vi "Map to Table.vi"(0 "Data":T1, 5 "error in":errorcluster) -> (14 "Value":string[][](array[string]), 19 "error out":errorcluster)   [LabVIEW 2024]
uses:
  Type Def/Data.ctl
panel:
  # "Connector Pane"
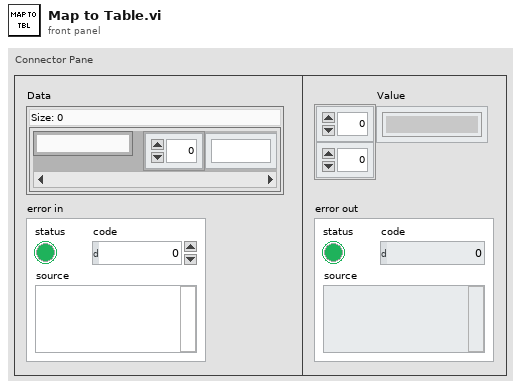
[diagram p1: front panel]
types:
  T1 = typedef "Data.ctl" = map{string, dbl[]}
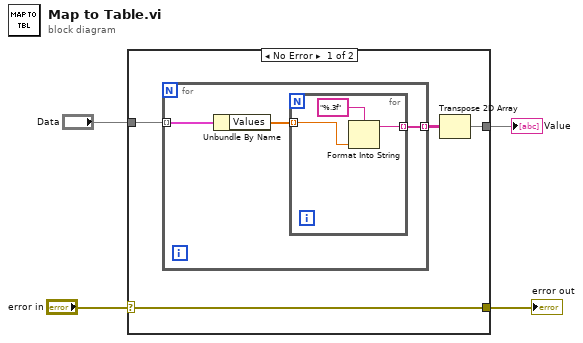
[diagram p0: block diagram]
diagram:
  n1 = case shown="No Error" "error in" {
    selector: "error in" -> [w6 w15]
    tunnel: [w6 w15] -> w3
    tunnel: "Data" -> [w8 _]
    tunnel: [w5 _] -> w1
    frame No Error {
      n2 = for {
        tunnel: w8 -> [w11] mode=indexing
        tunnel: [w9] -> w7 mode=indexing
        n3 = Unbundle By Name(w11) -> ("Values"=w10:dbl[])
        n4 = for {
          tunnel: w10 -> [w14] mode=indexing
          tunnel: [w12] -> w9 mode=indexing
          n5 = Format Into String(format string="%.3f", w14) -> (resulting string=w12:string)  [unwired: 2 in, 1 out]
        }
      }
      n6 = Transpose 2D Array(2D array=w7) -> (transposed array=w5:string[][])
    }
    frame Error {
    }
  }
  "error out" <- w3
  "Value" <- w1
